vi "hello World.vi"(11 "String":string="Hello World") -> ()   [LabVIEW 2019]
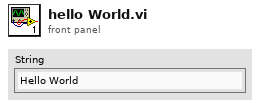
[diagram p1: front panel]
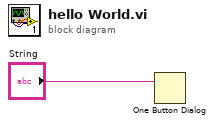
[diagram p0: block diagram]
diagram:
  n1 = One Button Dialog(message="String") -> ()  [unwired: 1 in, 1 out]
